vi "THzTimeAutoSave.vi"(5 "Autosave Directory for Long-term Average Scan":path, 6 "y-axis":dbl[](array[numeric]), 7 "x-axis":sgl[](array[numeric]), 8 "String":string, 9 "SaveFile name":string) -> ()   [LabVIEW 2010]
uses:
  <vilib>/Utility/file.llb/Write To Spreadsheet File (DBL).vi
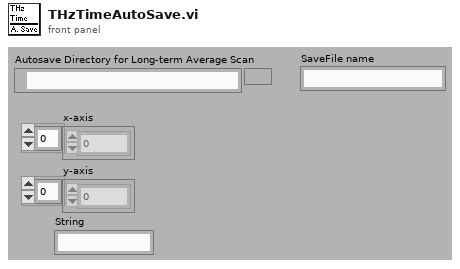
[diagram p1: front panel]
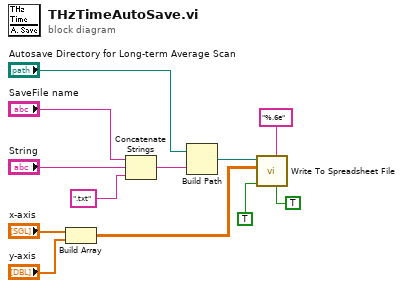
[diagram p0: block diagram]
diagram:
  n1 = Build Array("x-axis", "y-axis") -> (w11:dbl[][])
  n2 = Concatenate Strings("SaveFile name", "String", ".txt" ("string")) -> (w6:string)
  n3 = Build Path(base path="Autosave Directory for Long-term Average Scan", name or relative path=w6) -> (appended path=w12:path)
  n4 = call-poly <vilib>:"Write To Spreadsheet File.vi"("transpose? (no:F)"=TRUE ("transpose?\n(no:F)"), "format (%.3f)"="%.6e", "append to file? (new file:F)"=TRUE ("transpose?\n(no:F)"), "2D data"=w11, "file path (dialog if empty)"=w12) -> ()  [unwired: 3 in, 1 out]
